vi "New.vi"(8 "error in (no error)":errorcluster, 10 "Text":string="[LogFilterRules]\nGlobal.CSM = module1\nGlobal.CSM = module2\nGlobal.LogType = Status\nGlobal.State = Internal: Ignore1\nGlobal.StateType  = State - Internal State\npath = C:\\data\\\nabc = asvasdfsfasfasfasd\n        asdfdasfasdfasdf\n        123421423423432 \nmodule1.LogType = Status\nmodule1.LogType = Module Created\nmodule2.State = Internal: Ignore3\nmodule2.State = Internal: Ignore4\nmodule3.StateType  = State - Internal State", 11 "Path (\"\")":path=path "C:/Users/Supermanman/AppData/Local/Temp/lvtemporary_285019.ini") -> (0 "error out":errorcluster, 3 "LabVIEW-Config.lvlib:LabVIEW-Config.lvclass":refnum<class "LabVIEW-Config.lvclass">)   [LabVIEW 2017, in "LabVIEW-Config.lvlib" / "LabVIEW-Config.lvclass"]
uses:
  LabVIEW-Config.lvclass
  LineToken.ctl
  LabVIEW-Config.lvclass/LabVIEW-Config.ctl
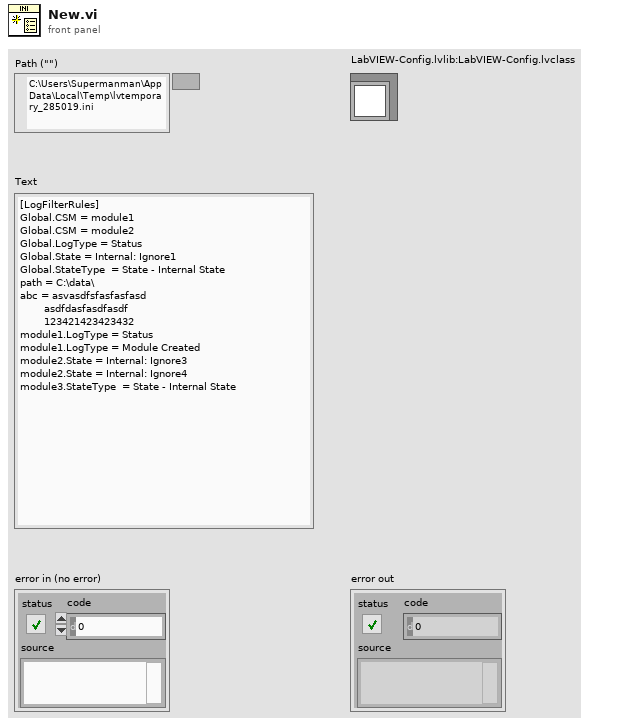
[diagram p1: front panel]
types:
  T1 = typedef "LabVIEW-Config.lvlib/LabVIEW-Config.lvclass/LineToken.ctl" = enum8{"comment", "section", "key", "more"}
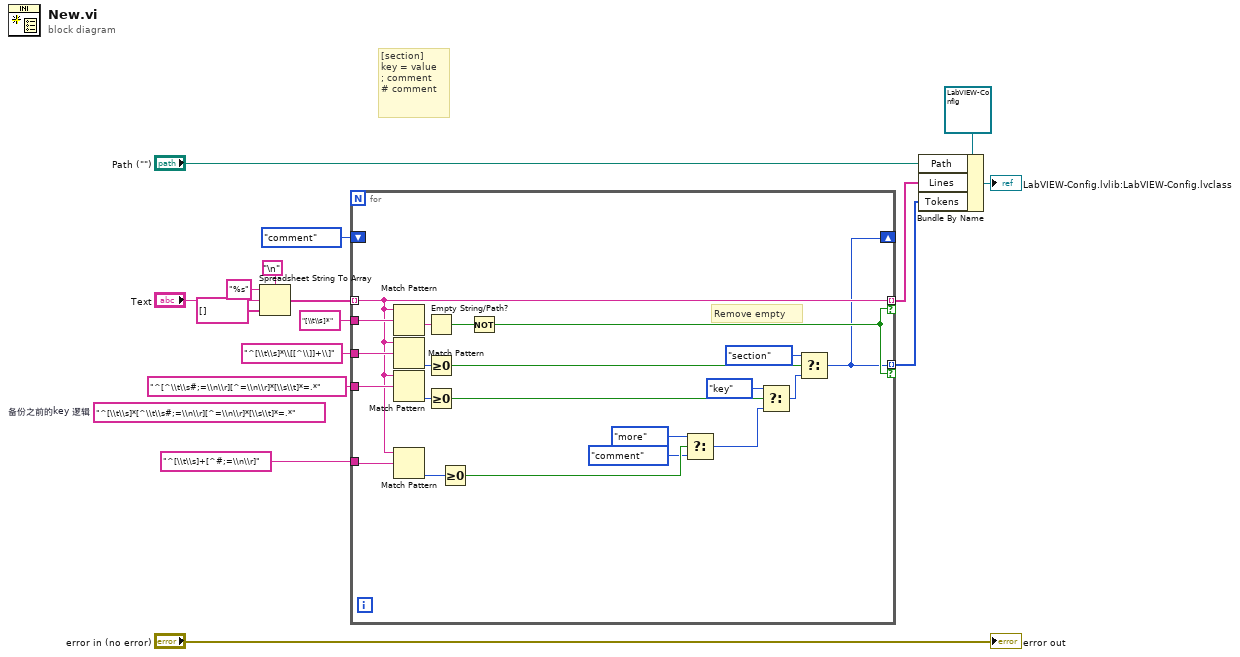
[diagram p0: block diagram]
diagram:
  (unwired) "^[\\t\\s]*[^\\t\\s#;=\\n\\r][^=\\n\\r]*[\\s\\t]*=.*"  # 备份之前的key 逻辑
  # "[section]\nkey = value\n; comment\n# comment"
  n1 = Spreadsheet String To Array(delimiter (Tab)="\n" ("Line Feed Constant"), format string="%s", spreadsheet string="Text", array type (2D Dbl)=string[] []) -> (array=w3:string[])
  n2 = for {
    tunnel: w3 -> [w22] mode=indexing
    tunnel: "^[\\t\\s]*\\[[^\\]]+\\]" ("regular expression") -> [w37]
    tunnel: [w17] -> w11 mode=indexing if=w30
    tunnel: "^[^\\t\\s#;=\\n\\r][^=\\n\\r]*[\\s\\t]*=.*" ("regular expression") -> [w32]
    tunnel: "[\\t\\s]*" ("regular expression") -> [w35]
    tunnel: [w22] -> w7 mode=indexing if=w30
    tunnel: "^[\\t\\s]+[^#;=\\n\\r]" ("regular expression") -> [w23]
    shift-right: [w17] -> _
    shift-left: LineToken."comment" ("Token") -> [_]
    # "Remove empty"
    n3 = Match Pattern(string=w22, regular expression=w35) -> (after substring=w36:string)  [unwired: 1 in, 3 out]
    n4 = Match Pattern(string=w22, regular expression=w37) -> (offset past match=w34:i32)  [unwired: 1 in, 3 out]
    n5 = Match Pattern(string=w22, regular expression=w32) -> (offset past match=w33:i32)  [unwired: 1 in, 3 out]
    n6 = Match Pattern(string=w22, regular expression=w23) -> (offset past match=w24:i32)  [unwired: 1 in, 3 out]
    n7 = Empty String/Path?(string/path=w36) -> (empty?=w31:bool)
    n8 = Greater Or Equal To 0?(x=w34) -> (x >= 0?=w29:bool)
    n9 = Greater Or Equal To 0?(x=w33) -> (x >= 0?=w25:bool)
    n10 = Greater Or Equal To 0?(x=w24) -> (x >= 0?=w21:bool)
    n11 = Not(x=w31) -> (.not. x?=w30:bool)
    n12 = Select(t=LineToken."more" ("Token"), s=w21, f=LineToken."comment" ("Token")) -> (s? t:f=w18:T1)
    n13 = Select(t=LineToken."key" ("Token"), s=w25, f=w18) -> (s? t:f=w26:T1)
    n14 = Select(t=LineToken."section" ("Token"), s=w29, f=w26) -> (s? t:f=w17:T1)
  }
  n15 = Bundle By Name(cluster=refnum<class "LabVIEW-Config.lvclass"> refnum ("Refnum"), "Path"="Path (\"\")", "Lines"=w7, "Tokens"=w11) -> (→"LabVIEW-Config.lvlib:LabVIEW-Config.lvclass":refnum<class "LabVIEW-Config.lvclass">)
  "error out" <- "error in (no error)"
